vi "CreateDataValidationFailureData.vi"(4 "RPM":sgl, 6 "SamplingInfo":cluster{"Fs":dbl, "#s":dbl}, 9 "in":waveform(dbl)[](array[waveform]), 10 "envelope signal amplitude":dbl=1.0 format="%#_13g", 11 "Value 2":T1(ring)) -> (1 "out":waveform(dbl)[](array[waveform]))   [LabVIEW 2017, in "CmsAcquisition.lvlib"]
uses:
  <vilib>/addons/InsightCM/Devices/Shared/Cms/CmsAcquisition/CmsAcquisition.lvlib
  <vilib>/measure/NI_MABase.lvlib
  <vilib>/addons/InsightCM/Utilities/Analysis/Vibration/VibrationAnalysisFunctions.lvlib
panel:
  out "Waveform Graph 2":cluster{"f0":dbl, "df":dbl, "magnitude":dbl[]}(graph)
  out "Waveform Graph":waveform(dbl)(graph)
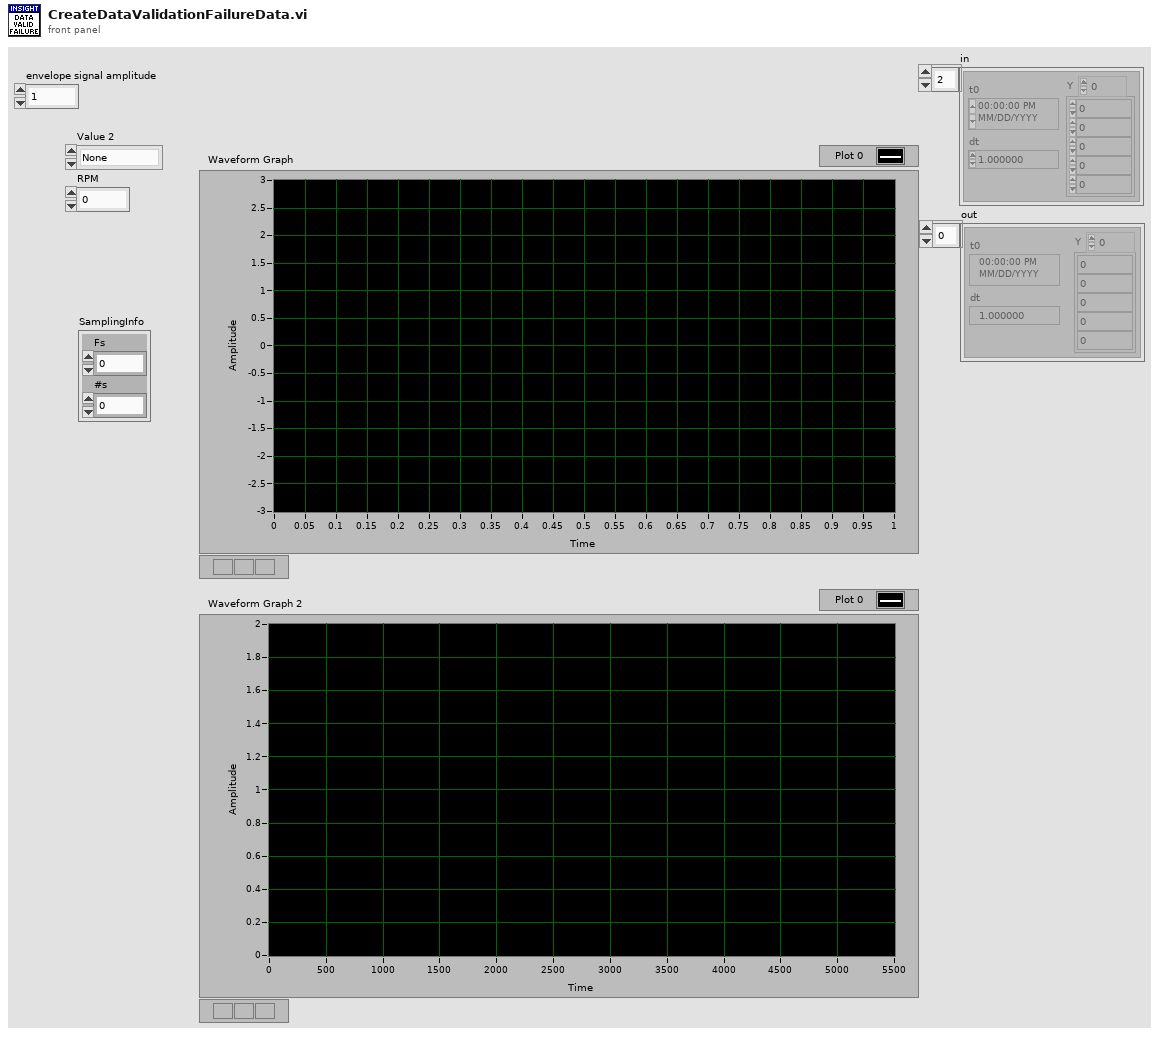
[diagram p1: front panel]
types:
  T1 = enum16{"None", "Pk_PkPK", "N Rule", "Z Rule", "U Rule", "Line Noise", "Low Signal", "Ski Slope", "Envelope Test"}
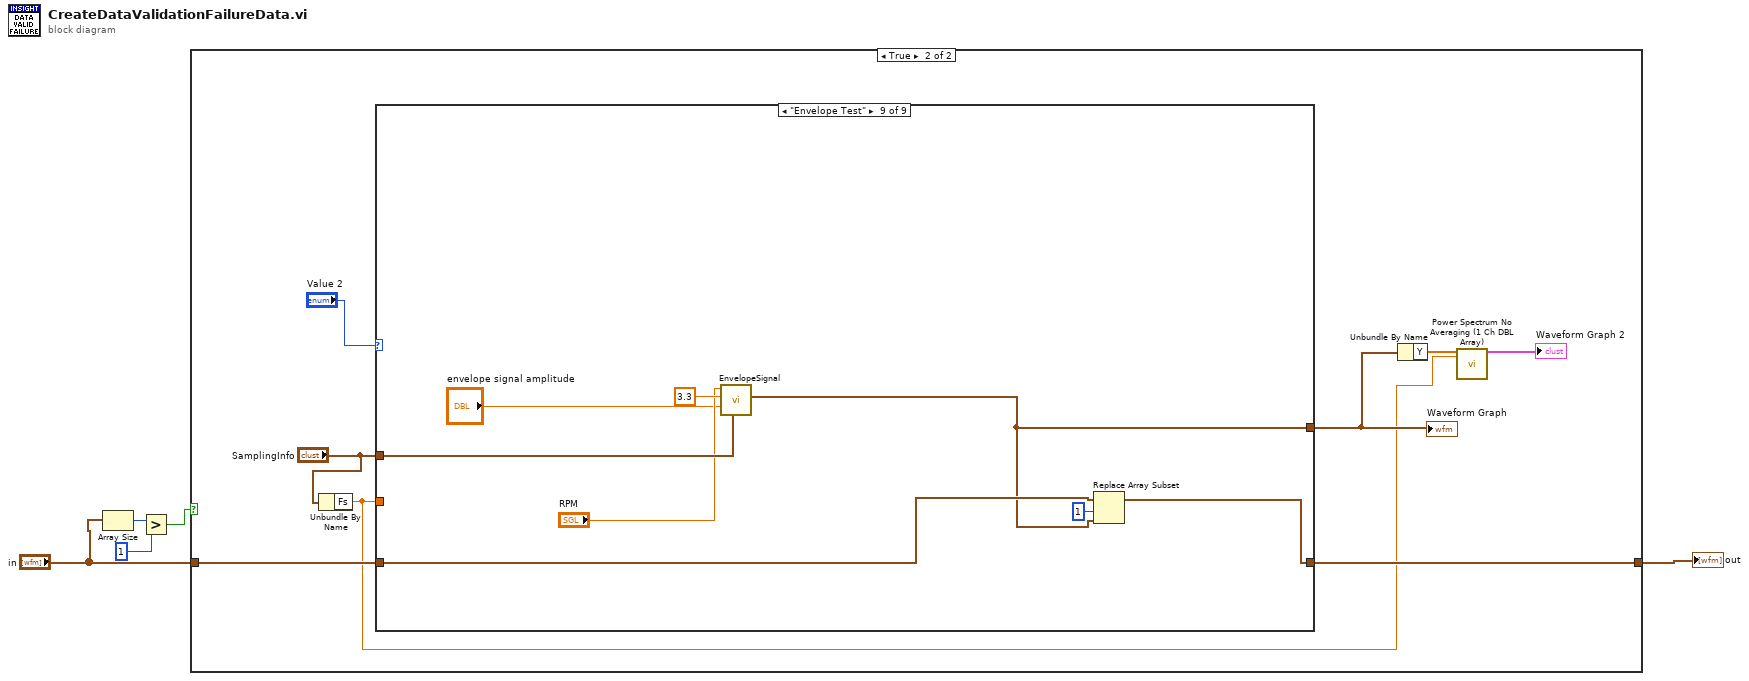
[diagram p0: block diagram]
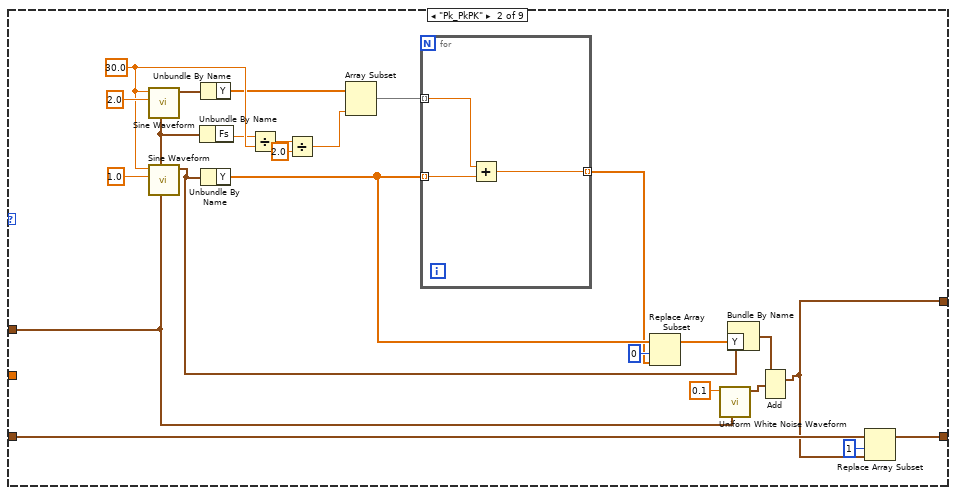
[diagram p4: hidden frame]
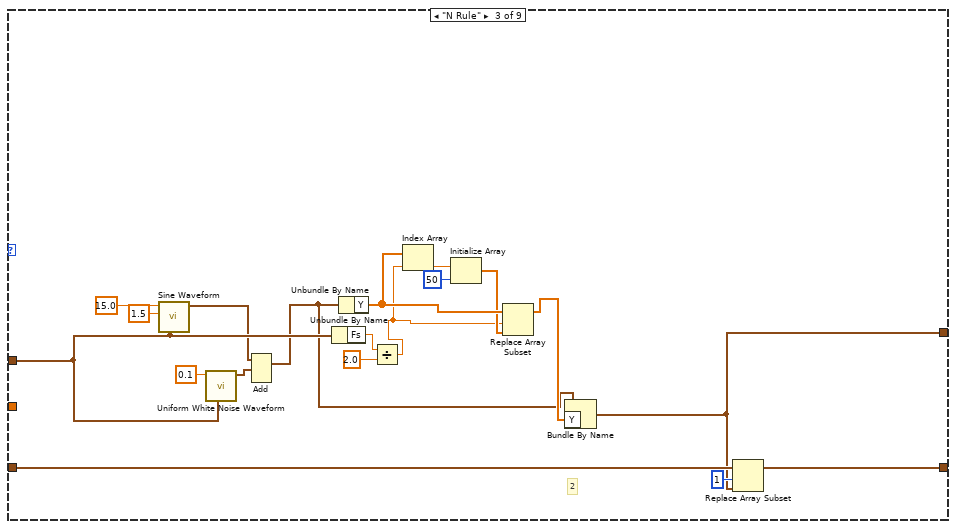
[diagram p5: hidden frame]
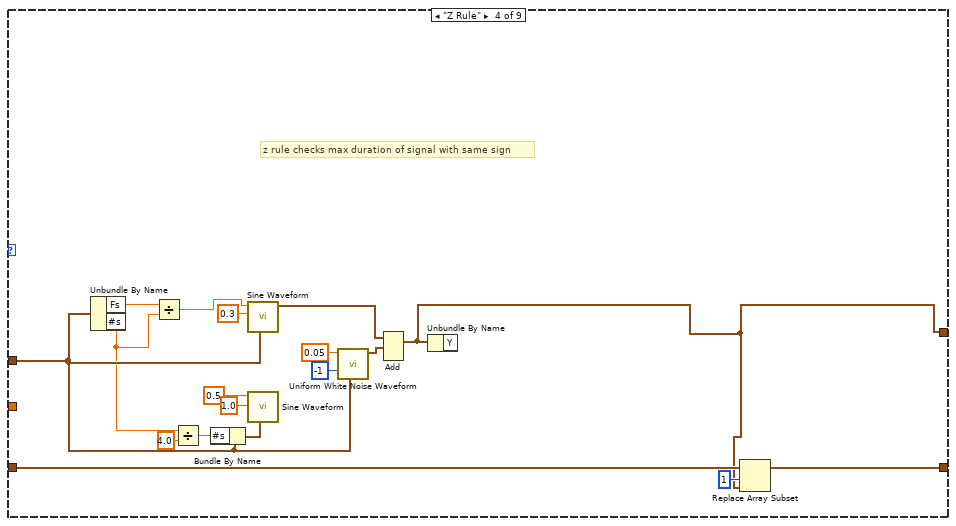
[diagram p6: hidden frame]
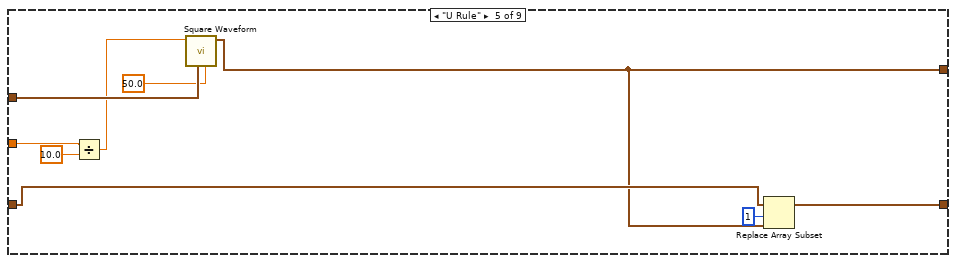
[diagram p7: hidden frame]
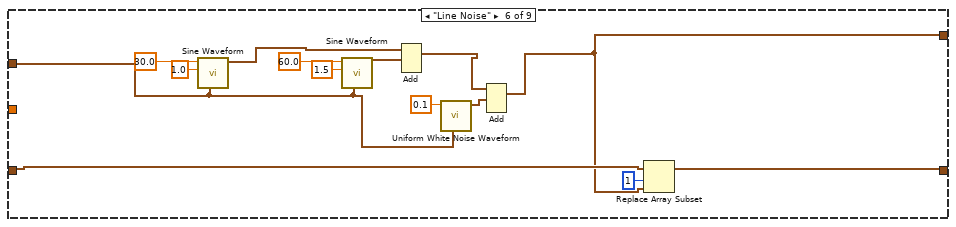
[diagram p8: hidden frame]
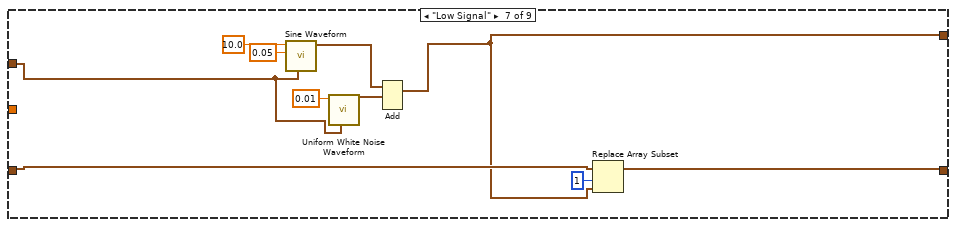
[diagram p9: hidden frame]
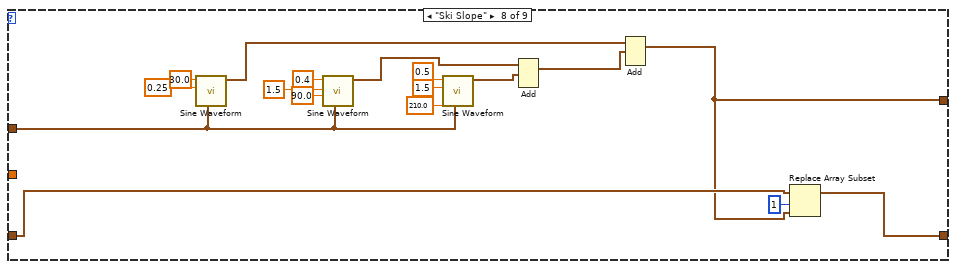
[diagram p10: hidden frame]
diagram:
  n1 = Array Size(array="in") -> (size(s)=w3:i32)
  n2 = Greater?(x=w3, y=1) -> (0:w1:bool)
  n3 = case shown="True" w1 {
    tunnel: "in" -> [w6 w14]
    tunnel: [w6 w13] -> w5
    frame False {
    }
    frame True {
      n4 = Unbundle By Name("SamplingInfo") -> ("Fs"=w7:dbl)
      n5 = case shown="\"Envelope Test\"" "Value 2" {
        tunnel: "SamplingInfo" -> [_ w18 w47 w70 w87 w91 w105 w126 w136]
        tunnel: [_ w16 w55 w61 w82 w88 w102 w113 w130] -> w9
        tunnel: [w15 w23 w56 w75 w84 w93 w107 w112 w131] -> w13
        tunnel: w14 -> [w15 w25 w57 w76 w83 w94 w108 w114 w132]
        tunnel: w7 -> [_ _ _ _ w81 _ _ _ _]
        frame "None", Default {
        }
        frame "Pk_PkPK" {
          w35 = 30.0 ("frequency")
          n6 = call <vilib>:"Sine Waveform.vi"("sampling info"=w18, "amplitude"=2.0, "frequency"=w35) -> ("signal out"=w36:waveform(dbl))  [unwired: 7 in, 1 out]
          n7 = call <vilib>:"Sine Waveform.vi"("sampling info"=w18, "amplitude"=1.0, "frequency"=w35) -> ("signal out"=w26:waveform(dbl))  [unwired: 7 in, 1 out]
          n8 = Unbundle By Name(w18) -> ("Fs"=w22:dbl)
          n9 = Unbundle By Name(w36) -> ("Y"=w32:dbl[])
          n10 = Unbundle By Name(w26) -> ("Y"=w29:dbl[])
          n11 = Divide(x=w22, y=w35) -> (x/y=w34:dbl)
          n12 = Divide(x=w34, y=2.0) -> (x/y=w31:dbl)
          n13 = Array Subset(array=w32, length=w31) -> (w30:dbl[])  [unwired: 1 in]
          n14 = for {
            tunnel: w30 -> [w40] mode=indexing
            tunnel: w29 -> [w41] mode=indexing
            tunnel: [w39] -> w27 mode=indexing
            n15 = Add(x=w40, y=w41) -> (x+y=w39:dbl)
          }
          n16 = Replace Array Subset(array=w29, new element=w27, index=0) -> (w21:dbl[])
          n17 = call <vilib>:"Uniform White Noise Waveform.vi"("sampling info"=w18, "amplitude"=0.1) -> ("signal out"=w20:waveform(dbl))  [unwired: 8 in, 1 out]
          n18 = Bundle By Name(cluster=w26, "Y"=w21) -> (w17:waveform(dbl))
          n19 = Add(1:w20, 2:w17) -> (0:w16:waveform(dbl))  [unwired: 1 in, 1 out]
          n20 = Replace Array Subset(array=w25, new element=w16, index=1) -> (w23:waveform(dbl)[])
        }
        frame "N Rule" {
          # "2"
          n21 = call <vilib>:"Sine Waveform.vi"("sampling info"=w47, "amplitude"=1.5, "frequency"=15.0) -> ("signal out"=w46:waveform(dbl))  [unwired: 7 in, 1 out]
          n22 = call <vilib>:"Uniform White Noise Waveform.vi"("sampling info"=w47, "amplitude"=0.1) -> ("signal out"=w49:waveform(dbl))  [unwired: 8 in, 1 out]
          n23 = Add(1:w49, 2:w46) -> (0:w45:waveform(dbl))  [unwired: 1 in, 1 out]
          n24 = Unbundle By Name(w47) -> ("Fs"=w44:dbl)
          n25 = Unbundle By Name(w45) -> ("Y"=w53:dbl[])
          n26 = Divide(x=w44, y=2.0) -> (x/y=w42:dbl)
          n27 = Index Array(array=w53, index=w42) -> (element=w52:dbl)
          n28 = Initialize Array(w52, 50 ("dimension size")) -> (w50:dbl[])
          n29 = Replace Array Subset(array=w53, new element=w50, index=w42) -> (w54:dbl[])
          n30 = Bundle By Name(cluster=w45, "Y"=w54) -> (w55:waveform(dbl))
          n31 = Replace Array Subset(array=w57, new element=w55, index=1) -> (w56:waveform(dbl)[])
        }
        frame "Z Rule" {
          # "z rule checks max duration of signal with same sign"
          n32 = Unbundle By Name(w70) -> ("Fs"=w66:dbl, "#s"=w65:dbl)
          n33 = Divide(x=w66, y=w65) -> (x/y=w64:dbl)
          n34 = Divide(x=w65, y=4.0) -> (x/y=w69:dbl)
          n35 = Bundle By Name(cluster=w70, "#s"=w69) -> (w68:cluster{"Fs":dbl, "#s":dbl})
          n36 = call <vilib>:"Sine Waveform.vi"("sampling info"=w70, "amplitude"=0.3, "frequency"=w64) -> ("signal out"=w62:waveform(dbl))  [unwired: 7 in, 1 out]
          n37 = call <vilib>:"Sine Waveform.vi"("sampling info"=w68, "amplitude"=1.0, "frequency"=0.5) -> ()  [unwired: 7 in, 2 out]
          n38 = call <vilib>:"Uniform White Noise Waveform.vi"("sampling info"=w70, "seed"=-1, "amplitude"=0.05) -> ("signal out"=w73:waveform(dbl))  [unwired: 7 in, 1 out]
          n39 = Add(1:w73, 2:w62) -> (0:w61:waveform(dbl))  [unwired: 1 in, 1 out]
          n40 = Unbundle By Name(w61) -> ()  [unwired: 1 out]
          n41 = Replace Array Subset(array=w76, new element=w61, index=1) -> (w75:waveform(dbl)[])
        }
        frame "U Rule" {
          n42 = Divide(x=w81, y=10.0) -> (x/y=w79:dbl)
          n43 = call <vilib>:"Square Waveform.vi"("duty cycle (%)"=50.0, "sampling info"=w87, "frequency"=w79) -> ("signal out"=w82:waveform(dbl))  [unwired: 7 in, 1 out]
          n44 = Replace Array Subset(array=w83, new element=w82, index=1) -> (w84:waveform(dbl)[])
        }
        frame "Line Noise" {
          n45 = call <vilib>:"Sine Waveform.vi"("sampling info"=w91, "amplitude"=1.0, "frequency"=30.0) -> ("signal out"=w96:waveform(dbl))  [unwired: 7 in, 1 out]
          n46 = call <vilib>:"Sine Waveform.vi"("sampling info"=w91, "amplitude"=1.5, "frequency"=60.0) -> ("signal out"=w97:waveform(dbl))  [unwired: 7 in, 1 out]
          n47 = Add(1:w97, 2:w96) -> (0:w89:waveform(dbl))  [unwired: 1 in, 1 out]
          n48 = call <vilib>:"Uniform White Noise Waveform.vi"("sampling info"=w91, "amplitude"=0.1) -> ("signal out"=w92:waveform(dbl))  [unwired: 8 in, 1 out]
          n49 = Add(1:w92, 2:w89) -> (0:w88:waveform(dbl))  [unwired: 1 in, 1 out]
          n50 = Replace Array Subset(array=w94, new element=w88, index=1) -> (w93:waveform(dbl)[])
        }
        frame "Low Signal" {
          n51 = call <vilib>:"Sine Waveform.vi"("sampling info"=w105, "amplitude"=0.05, "frequency"=10.0) -> ("signal out"=w103:waveform(dbl))  [unwired: 7 in, 1 out]
          n52 = call <vilib>:"Uniform White Noise Waveform.vi"("sampling info"=w105, "amplitude"=0.01) -> ("signal out"=w104:waveform(dbl))  [unwired: 8 in, 1 out]
          n53 = Add(1:w104, 2:w103) -> (0:w102:waveform(dbl))  [unwired: 1 in, 1 out]
          n54 = Replace Array Subset(array=w108, new element=w102, index=1) -> (w107:waveform(dbl)[])
        }
        frame "Ski Slope" {
          n55 = call <vilib>:"Sine Waveform.vi"("sampling info"=w126, "amplitude"=0.25, "frequency"=30.0) -> ("signal out"=w119:waveform(dbl))  [unwired: 7 in, 1 out]
          n56 = call <vilib>:"Sine Waveform.vi"("sampling info"=w126, "phase"=90.0, "amplitude"=1.5, "frequency"=0.4) -> ("signal out"=w117:waveform(dbl))  [unwired: 6 in, 1 out]
          n57 = call <vilib>:"Sine Waveform.vi"("sampling info"=w126, "phase"=210.0, "amplitude"=1.5, "frequency"=0.5) -> ("signal out"=w118:waveform(dbl))  [unwired: 6 in, 1 out]
          n58 = Add(1:w118, 2:w117) -> (0:w116:waveform(dbl))  [unwired: 1 in, 1 out]
          n59 = Add(1:w116, 2:w119) -> (0:w113:waveform(dbl))  [unwired: 1 in, 1 out]
          n60 = Replace Array Subset(array=w114, new element=w113, index=1) -> (w112:waveform(dbl)[])
        }
        frame "Envelope Test" {
          n61 = call <vilib>:"EnvelopeSignal.vi"("sampling info"=w136, "amplitude"="envelope signal amplitude", "Fault (order)"=3.3, "Running Speed (RPM)"="RPM") -> ("Waveform"=w130:waveform(dbl))  [unwired: 4 in, 3 out]
          n62 = Replace Array Subset(array=w132, new element=w130, index=1) -> (w131:waveform(dbl)[])
        }
      }
      "Waveform Graph" <- w9
      n63 = Unbundle By Name(w9) -> ("Y"=w11:dbl[])
      n64 = call <vilib>:"Power Spectrum No Averaging (1 Ch DBL Array).vi"("scaled signal [EU]"=w11, "sampling rate [Hz]"=w7) -> ("power spectrum [EU^2 rms]"=→"Waveform Graph 2":cluster{"f0":dbl, "df":dbl, "magnitude":dbl[]})  [unwired: 16 in, 1 out]
    }
  }
  "out" <- w5
